vi "SCD Range Mode.vi"(11 "error in":errorcluster) -> (15 "error out":errorcluster)   [LabVIEW 2020, in "Examples.lvlib"]
doc: "Example for a SCD spectrum acquisition."
uses:
  Examples.lvlib
  Classes/SCD/acqSet.ctl
  2c696148-80e0-4d05-9eda-620825821f52.vi
  9b69558d-0271-42a7-9057-1b73895216a6.vi
  efc0c87d-66c5-4069-95b0-7601b8aa1897.vi
  30aba31c-a5e2-4a44-8a7d-d1cf740afd9f.vi
  Classes/Mono/Monochromator.lvclass
  Classes/SCD/SCD.lvclass
panel:
  in  "wavelengths to cover":dbl[](array[numeric])=[500.0, 505.0, 510.0]
  out "isBusy":bool
  out "isDataAvailable?":bool
  # "Connector Pane"
  # "Locals"
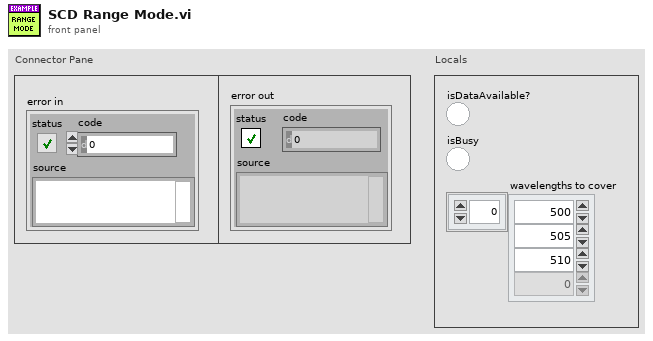
[diagram p1: front panel]
types:
  T1 = typedef "horiba.lvlib/SCD.lvclass/acqSet.ctl" = cluster{"scanCount":i32, "timeStep":i32, "integrationTime":i32, "externalParam":i32}
  T2 = cluster{"currentSignal":cluster{"unit":string, "value":dbl}, "elapsedTime":dbl, "event_marker":bool, "overscale_current_channel":bool, "overscale_voltage_channel":bool, "pmtSignal":cluster{"unit":string, "value":dbl}, "pointNumber":dbl, "ppdSignal":cluster{"unit":string, "value":dbl}, "voltageSignal":cluster{"unit":string, "value":dbl}}[]
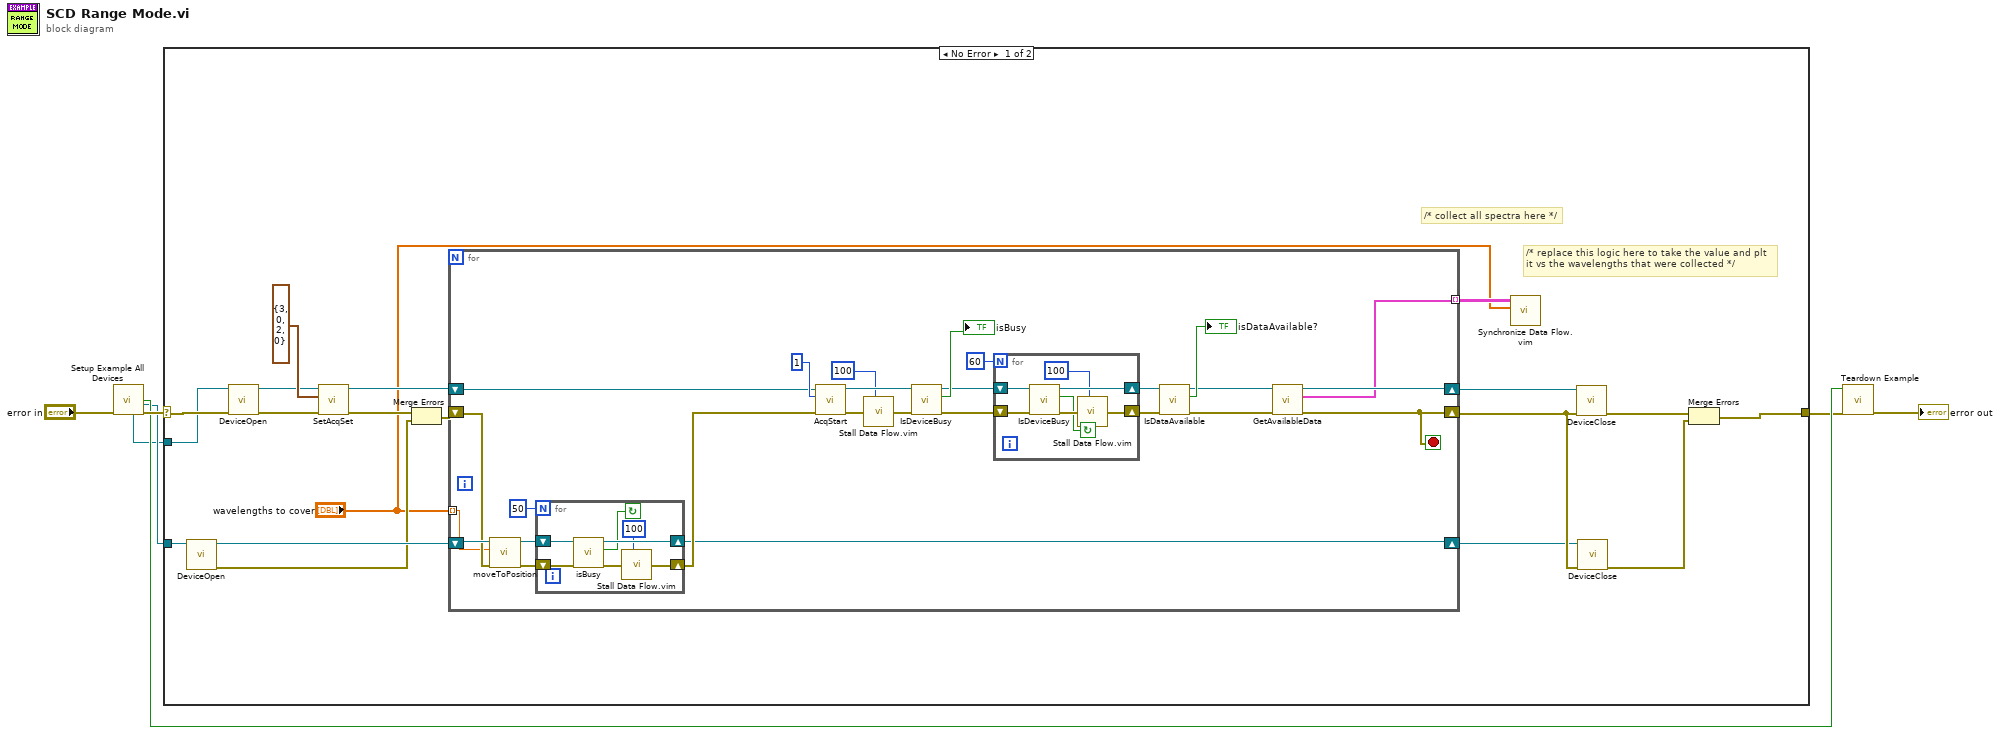
[diagram p0: block diagram]
diagram:
  n1 = call "Setup Example All Devices.vi"("error in (no error)"="error in") -> ("error out"=w5:errorcluster, "Mono out"=w2:refnum<class "Monochromator.lvclass">, "Module Was Already Running?"=w4:bool, "SCD out"=w1:refnum<class "SCD.lvclass">)  [unwired: 6 in, 1 out]
  n2 = case shown="No Error" w5 {
    selector: w5 -> [w16 w67]
    tunnel: [w18 w67] -> w3
    tunnel: w2 -> [w24 _]
    tunnel: w1 -> [w9 _]
    frame No Error {
      # "/* replace this logic here to take the value and plt\nit vs the wavelengths that were collected */"
      # "/* collect all spectra here */"
      n3 = call-dynamic "DeviceOpen.vi"("Monochromator in"=w24) -> ("error out"=w21:errorcluster, "Monochromator out"=w23:refnum<class "Monochromator.lvclass">)  [unwired: 7 in, 2 out]
      n4 = call-dynamic "DeviceOpen.vi"("error in (no error)"=w16, "SCD in"=w9) -> ("error out"=w10:errorcluster, "SCD out"=w8:refnum<class "SCD.lvclass">)  [unwired: 6 in, 2 out]
      n5 = call "SetAcqSet.vi"("error in (no error)"=w10, "integration_time"=T1 {"scanCount"=3, "timeStep"=0, "integrationTime"=2, "externalParam"=0}, "SCD in"=w8) -> ("error out"=w14:errorcluster, "SCD out"=w15:refnum<class "SCD.lvclass">)  [unwired: 7 in]
      n6 = Merge Errors(w14, w21) -> (w22:errorcluster)
      n7 = for {
        shift-right: [w28] -> w20
        shift-left: w22 -> [w43]
        shift-right: [w33] -> w25
        shift-left: w15 -> [w27]
        shift-right: [w30] -> w19
        shift-left: w23 -> [w44]
        tunnel: [w32] -> w13 mode=indexing
        tunnel: "wavelengths to cover" -> [w31] mode=indexing
        stop <- w28 stop-if-true
        n8 = call "moveToPosition.vi"("error in (no error)"=w43, "wavelength"=w31, "Monochromator in"=w44) -> ("error out"=w47:errorcluster, "Monochromator out"=w46:refnum<class "Monochromator.lvclass">)  [unwired: 5 in, 2 out]
        n9 = for {
          N: 50 -> [_]
          shift-right: [w62] -> w34
          shift-left: w47 -> [w66]
          shift-right: [w63] -> w30
          shift-left: w46 -> [w64]
          stop <- w60 continue-if-true
          n10 = call "isBusy.vi"("error in (no error)"=w66, "Monochromator in"=w64) -> ("error out"=w65:errorcluster, "mono is busy?"=w60:bool, "Monochromator out"=w63:refnum<class "Monochromator.lvclass">)  [unwired: 7 in]
          n11 = call "Stall Data Flow.vim"("value in"=w65, "milliseconds to wait"=u32 100) -> ("value out"=w62:errorcluster)  [unwired: 1 out]
        }
        n12 = call "AcqStart.vi"("error in (no error)"=w34, "trigger"=1, "SCD in"=w27) -> ("error out"=w52:errorcluster, "SCD out"=w51:refnum<class "SCD.lvclass">)  [unwired: 7 in]
        n13 = call "Stall Data Flow.vim"("value in"=w52, "milliseconds to wait"=u32 100) -> ("value out"=w50:errorcluster)  [unwired: 1 out]
        n14 = call "IsDeviceBusy.vi"("error in (no error)"=w50, "SCD in"=w51) -> ("error out"=w35:errorcluster, "isBusy"=→"isBusy":bool, "SCD out"=w36:refnum<class "SCD.lvclass">)  [unwired: 7 in]
        n15 = for {
          N: 60 -> [_]
          shift-right: [w58] -> w40
          shift-left: w36 -> [w59]
          shift-right: [w54] -> w41
          shift-left: w35 -> [w57]
          stop <- w55 continue-if-true
          n16 = call "IsDeviceBusy.vi"("error in (no error)"=w57, "SCD in"=w59) -> ("error out"=w56:errorcluster, "isBusy"=w55:bool, "SCD out"=w58:refnum<class "SCD.lvclass">)  [unwired: 7 in]
          n17 = call "Stall Data Flow.vim"("value in"=w56, "milliseconds to wait"=u32 100) -> ("value out"=w54:errorcluster)  [unwired: 1 out]
        }
        n18 = call "IsDataAvailable.vi"("error in (no error)"=w41, "SCD in"=w40) -> ("error out"=w38:errorcluster, "isDataAvailable?"=→"isDataAvailable?":bool, "SCD out"=w39:refnum<class "SCD.lvclass">)  [unwired: 7 in]
        n19 = call "GetAvailableData.vi"("error in (no error)"=w38, "SCD in"=w39) -> ("error out"=w28:errorcluster, "data"=w32:T2, "SCD out"=w33:refnum<class "SCD.lvclass">)  [unwired: 7 in]
      }
      n20 = call "Synchronize Data Flow.vim"("input 2"="wavelengths to cover", "input 1"=w13) -> ()  [unwired: 2 in, 4 out]
      n21 = call-dynamic "DeviceClose.vi"("error in (no error)"=w20, "SCD in"=w25) -> ("error out"=w26:errorcluster)  [unwired: 5 in, 4 out]
      n22 = call-dynamic "DeviceClose.vi"("error in (no error)"=w20, "Monochromator in"=w19) -> ("error out"=w17:errorcluster)  [unwired: 5 in, 4 out]
      n23 = Merge Errors(w26, w17) -> (w18:errorcluster)
    }
    frame Error {
    }
  }
  n24 = call "Teardown Example.vi"("error in (no error)"=w3, "Module Was Already Running?"=w4) -> ("error out"=→"error out":errorcluster)  [unwired: 9 in]
